vi "GetBlueSerialVirtualFolder.vi"(8 "error in (no error)":errorcluster, 10 "Virtual Folder":T1, 11 "LVClassLibrary Ref":refnum<vi>) -> (0 "error out":errorcluster, 2 "Folder Refnum out":refnum<vi>, 3 "LVClassLibrary Ref":refnum<vi>)   [LabVIEW 2019, in "BlueSerializationScripts.lvlib"]
uses:
  BlueSerializationScripts.lvlib
  BlueSerialVirtualFolders.ctl
  c83b021a-389f-4a7d-992f-795e26e2f350.vi
  91af645b-5fd7-4597-bd96-0d9170c3029d.vi
  70282a4b-f3c7-403f-adca-e8901aa301fb.vi
  c83b021a-389f-4a7d-992f-795e26e2f350.vi/fdedc02e-b8df-4f5c-a67d-f7a054b0afc0.vi
  91af645b-5fd7-4597-bd96-0d9170c3029d.vi/7f39a406-ba4d-436b-8f4c-8b55360affbf.vi
  70282a4b-f3c7-403f-adca-e8901aa301fb.vi/9e731682-4e33-4b2d-a7fb-c234dd1053df.vi
  BlueSerialProviderGlobal.vi
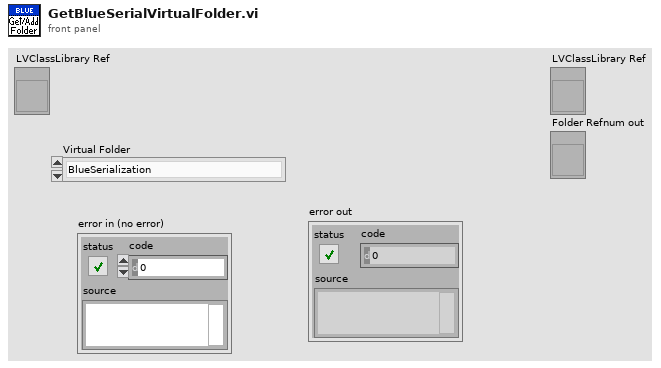
[diagram p1: front panel]
types:
  T1 = typedef "BlueSerializationScripts.lvlib/BlueSerialVirtualFolders.ctl" = enum16{"BlueSerialization", "Mutations"}
  T2 = enum32{"invalid scope", "public", "private", "protected", "community"}
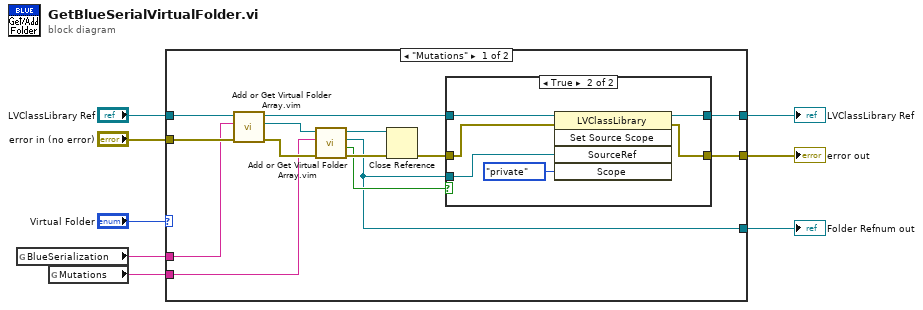
[diagram p0: block diagram]
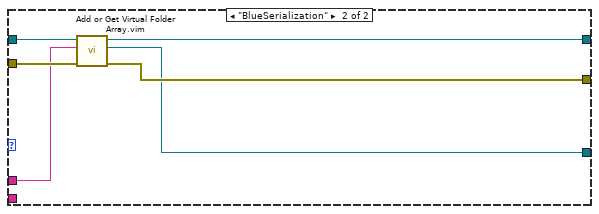
[diagram p3: hidden frame]
diagram:
  n1 = global read "BlueSerialProviderGlobal.vi" "BlueSerialization"() -> (w8:string)
  n2 = global read "BlueSerialProviderGlobal.vi" "Mutations"() -> (w7:string)
  n3 = case shown="\"Mutations\"" "Virtual Folder" {
    tunnel: w8 -> [w17 w32]
    tunnel: w7 -> [w15 _]
    tunnel: "LVClassLibrary Ref" -> [w19 w36]
    tunnel: "error in (no error)" -> [w18 w35]
    tunnel: [w10 w31] -> w2
    tunnel: [w9 w33] -> w3
    tunnel: [w12 w34] -> w1
    frame "Mutations" {
      n4 = call "Add or Get Virtual Folder Array.vim"("error in (no error)"=w18, "Virtual Folder Name"=w17, "ProjectItem"=w19) -> ("error out"=w22:errorcluster, "Folder Refnum out"=w16:refnum<vi>, "ProjectItem"=w13:refnum<vi>)  [unwired: 5 in, 1 out]
      n5 = call "Add or Get Virtual Folder Array.vim"("error in (no error)"=w22, "Virtual Folder Name"=w15, "ProjectItem"=w16) -> ("error out"=w20:errorcluster, "folder created?"=w14:bool, "Folder Refnum out"=w10:refnum<vi>, "ProjectItem"=w21:refnum<vi>)  [unwired: 5 in]
      n6 = Close Reference(reference=w21, error in (no error)=w20) -> (error out=w11:errorcluster)
      n7 = case shown="True" w14 {
        tunnel: w10 -> [_ w28]
        tunnel: w13 -> [w24 w30]
        tunnel: [w24 w29] -> w12
        tunnel: w11 -> [w23 w26]
        tunnel: [w23 w25] -> w9
        frame False {
        }
        frame True {
          n8 = invoke class="LVClassLibrary" method="Set Source Scope"(reference=w30, error in=w26, "SourceRef"=w28, "Scope"=T2."private" ("scope")) -> (reference out=w29:refnum<vi>, error out=w25:errorcluster)  [unwired: 1 in, 3 out]
        }
      }
    }
    frame "BlueSerialization" {
      n9 = call "Add or Get Virtual Folder Array.vim"("error in (no error)"=w35, "Virtual Folder Name"=w32, "ProjectItem"=w36) -> ("error out"=w33:errorcluster, "Folder Refnum out"=w31:refnum<vi>, "ProjectItem"=w34:refnum<vi>)  [unwired: 5 in, 1 out]
    }
  }
  "error out" <- w3
  "LVClassLibrary Ref" <- w1
  "Folder Refnum out" <- w2
